vi "ADC AI Global.vi"() -> ()   [LabVIEW 2013]
panel:
  out "AI16-47":fxp<+/-,28,17>[](array[numeric])
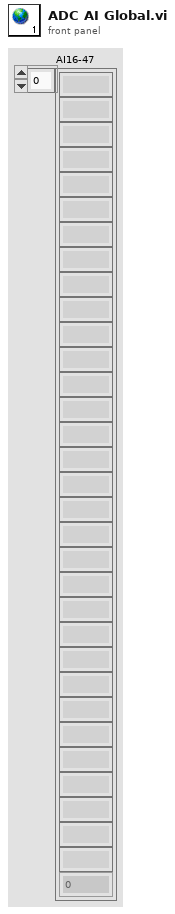
[diagram p1: front panel]
diagram:
